vi "Do HTML Async.vi"(7 "VolatusAPI":refnum<class "VolatusAPI.lvclass">, 10 "Value":bool, 11 "HtmlButtonControl in":refnum<class "HttpButtonControl.lvclass">) -> ()   [LabVIEW 2020, in "VolatusGUIElements.lvlib" / "HttpButtonControl.lvclass"]
uses:
  HttpButtonControl.lvclass
  Volatus/VolatusAPI/VolatusAPI.lvclass
  HttpButtonControl.lvclass/HttpButtonControl.ctl
  <vilib>/httpClient/LabVIEWHTTPClient.lvlib
  <vilib>/httpClient/POSTBuffer.vi
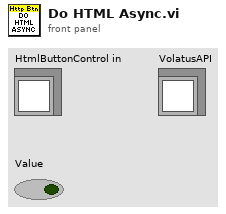
[diagram p1: front panel]
types:
  T1 = typedef "VolatusGUIElements.lvlib/HttpButtonControl.lvclass/Method.ctl" = enum16{"Get", "Post"}
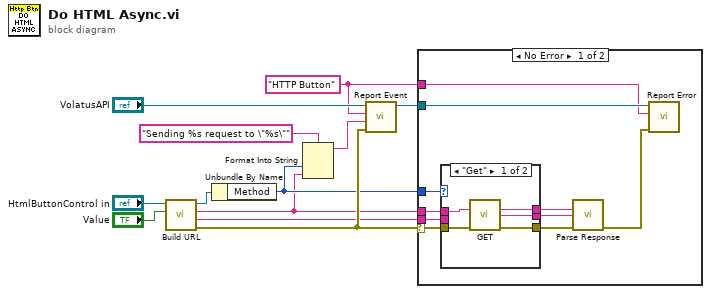
[diagram p0: block diagram]
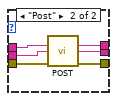
[diagram p2: hidden frame]
diagram:
  w1 = "HTTP Button" ("Context")
  n1 = call "Build URL.vi"("Value"="Value", "HttpButtonControl in"="HtmlButtonControl in") -> ("error out"=w6:errorcluster, "Post Buffer"=w3:string, "URL"=w4:string, "HttpButtonControl out"=w10:refnum<class "HttpButtonControl.lvclass">)  [unwired: 6 in]
  n2 = Unbundle By Name(w10) -> ("Method"=w5:T1)
  n3 = Format Into String(format string="Sending %s request to \"%s\"", w5, w4) -> (resulting string=w7:string)  [unwired: 2 in, 1 out]
  n4 = call "Report Event.vi"("error in (no error)"=w6, "Message"=w7, "Context"=w1, "VolatusAPI in"="VolatusAPI") -> ("VolatusAPI out"=w2:refnum<class "VolatusAPI.lvclass">)  [unwired: 6 in, 1 out]
  n5 = case shown="No Error" w6 {
    selector: w6 -> [w21 _]
    tunnel: w5 -> [w22 _]
    tunnel: w4 -> [w20 _]
    tunnel: w3 -> [w19 _]
    tunnel: w2 -> [w18 _]
    tunnel: w1 -> [w16 _]
    frame No Error {
      n6 = case shown="\"Get\"" w22 {
        tunnel: w21 -> [w27 w33]
        tunnel: w20 -> [w26 w31]
        tunnel: w19 -> [_ w32]
        tunnel: [w25 w30] -> w17
        tunnel: [w23 w29] -> w14
        tunnel: [w24 w28] -> w13
        frame "Get" {
          n7 = call <vilib>:"GET.vi"("url"=w26, "error in (no error)"=w27) -> ("headers"=w24:string, "body"=w23:string, "error out"=w25:errorcluster)  [unwired: 10 in, 1 out]
        }
        frame "Post" {
          n8 = call-poly <vilib>:"POST.vi"("url"=w31, "buffer"=w32, "error in (no error)"=w33) -> ("headers"=w28:string, "body"=w29:string, "error out"=w30:errorcluster)  [unwired: 9 in, 1 out]
        }
      }
      n9 = call "Parse Response.vi"("Headers"=w13, "Body"=w14, "error in (no error)"=w17) -> ("error out"=w15:errorcluster)  [unwired: 11 in, 1 out]
      n10 = call "Report Error.vi"("error in (no error)"=w15, "Context"=w16, "VolatusAPI in"=w18) -> ()  [unwired: 7 in, 2 out]
    }
    frame Error {
    }
  }
